vi "KeyDown.vi"(6 "PlatMods":T9, 7 "Type":T1, 8 "error in (no error)":errorcluster, 9 "VKey":T10, 10 "Char":i16, 11 "Data in":T2={"Class"={"Ants"=refnum, "Layer"=refnum, "Templates"=refnum, "Icon"=refnum, "Glyph"=refnum, "Settings"=refnum, "Tools"=refnum, "History"=refnum}, "Ref"={"Add Layer"=refnum, "Remove Layer"=refnum, "Line Text"=[], "Body Text Spec"=refnum, "DNL_Font"=refnum, "glyph path str"=refnum, "templates path str"=refnum, "Arrow Up"=refnum, "Arrow Down"=refnum, "IE VI Ref"=refnum, "Glyphs tree"=refnum, "Templates tree"=refnum, "Layer Icon Text"=refnum, "Layer Template"=refnum, "Body Text"=refnum, "Search Templates"=refnum, "TextMarker"=refnum, "Tab Control"=refnum, "Search Glyphs"=refnum, "Line Color"=refnum, "DNL_Glyphs []"=refnum, "Fill Color"=refnum, "Tools"=refnum, "Icon"=refnum, "Preview"=refnum, "Ants"=refnum, "Terminals"=refnum, "menu reference"=refnum, "LayerNames"=[], "GlyphLoadAnimation"=refnum, "TemplateLoadAnimation"=refnum, "refreshGlyphs"=refnum, "refreshTemplates"=refnum}, "Support"={"AntsRect"={"left"=0, "top"=0, "right"=0, "bottom"=0}, "Mouse Move Coords"={"Horizontal"=0, "Vertical"=0}, "Mouse Down Coords"={"Horizontal"=0, "Vertical"=0}, "Temp Coord"={"Horizontal"=0, "Vertical"=0}, "Action"=enum."Default", "Edge Color"=4914962, "Fill Color"=16860, "Mouse Down?"=FALSE, "Draft Mode?"=FALSE, "Temp Icon"=bytes[3102], "CTRL Pressed"=FALSE, "Move Selection?"=FALSE, "AntsRect Orig"={"left"=0, "top"=0, "right"=0, "bottom"=0}, "Text"="", "TM Set?"=FALSE, "Mouse inside icon?"=FALSE, "Tool (old value)"=0, "Pencil Move Color"=0, "Swap Colors?"=FALSE, "Shift pressed?"=FALSE}}) -> (0 "error out":errorcluster, 1 "Discard?":bool, 3 "Data out":T2={"Class"={"Ants"=refnum, "Layer"=refnum, "Templates"=refnum, "Icon"=refnum, "Glyph"=refnum, "Settings"=refnum, "Tools"=refnum, "History"=refnum}, "Ref"={"Add Layer"=refnum, "Remove Layer"=refnum, "Line Text"=[], "Body Text Spec"=refnum, "DNL_Font"=refnum, "glyph path str"=refnum, "templates path str"=refnum, "Arrow Up"=refnum, "Arrow Down"=refnum, "IE VI Ref"=refnum, "Glyphs tree"=refnum, "Templates tree"=refnum, "Layer Icon Text"=refnum, "Layer Template"=refnum, "Body Text"=refnum, "Search Templates"=refnum, "TextMarker"=refnum, "Tab Control"=refnum, "Search Glyphs"=refnum, "Line Color"=refnum, "DNL_Glyphs []"=refnum, "Fill Color"=refnum, "Tools"=refnum, "Icon"=refnum, "Preview"=refnum, "Ants"=refnum, "Terminals"=refnum, "menu reference"=refnum, "LayerNames"=[], "GlyphLoadAnimation"=refnum, "TemplateLoadAnimation"=refnum, "refreshGlyphs"=refnum, "refreshTemplates"=refnum}, "Support"={"AntsRect"={"left"=0, "top"=0, "right"=0, "bottom"=0}, "Mouse Move Coords"={"Horizontal"=0, "Vertical"=0}, "Mouse Down Coords"={"Horizontal"=0, "Vertical"=0}, "Temp Coord"={"Horizontal"=0, "Vertical"=0}, "Action"=enum."Default", "Edge Color"=4914962, "Fill Color"=16860, "Mouse Down?"=FALSE, "Draft Mode?"=FALSE, "Temp Icon"=bytes[3102], "CTRL Pressed"=FALSE, "Move Selection?"=FALSE, "AntsRect Orig"={"left"=0, "top"=0, "right"=0, "bottom"=0}, "Text"="", "TM Set?"=FALSE, "Mouse inside icon?"=FALSE, "Tool (old value)"=0, "Pencil Move Color"=0, "Swap Colors?"=FALSE, "Shift pressed?"=FALSE}})   [LabVIEW 2020]
uses:
  Class/Ants/Ants.lvclass
  Class/FakedArray/FakedArray.lvclass
  vi.lib/LabVIEW Icon API/lv_icon/Classes/Icon/Icon.lvclass
  Class/Icon Library/Glyph.lvclass
  Class/Settings/Settings.lvclass
  Class/Tools/Tools Paint.lvclass
  lv_icon.lvlib
  <vilib>/Utility/miscctls.llb/LVPoint32TypeDef.ctl
  <vilib>/event_ctls.llb/lveventtype.ctl
  Controls/SupportClass_Action.ctl
  <vilib>/event_ctls.llb/eventvkey.ctl
  Controls/Support Cluster.ctl
  Controls/References Cluster.ctl
  Controls/IE Classes.ctl
  Controls/Global Data.ctl
  vi.lib/LabVIEW Icon API/lv_icon/Controls/IEColor.ctl
  History/History/History.lvclass
panel:
  in  "Layer name":string="Clipboard"
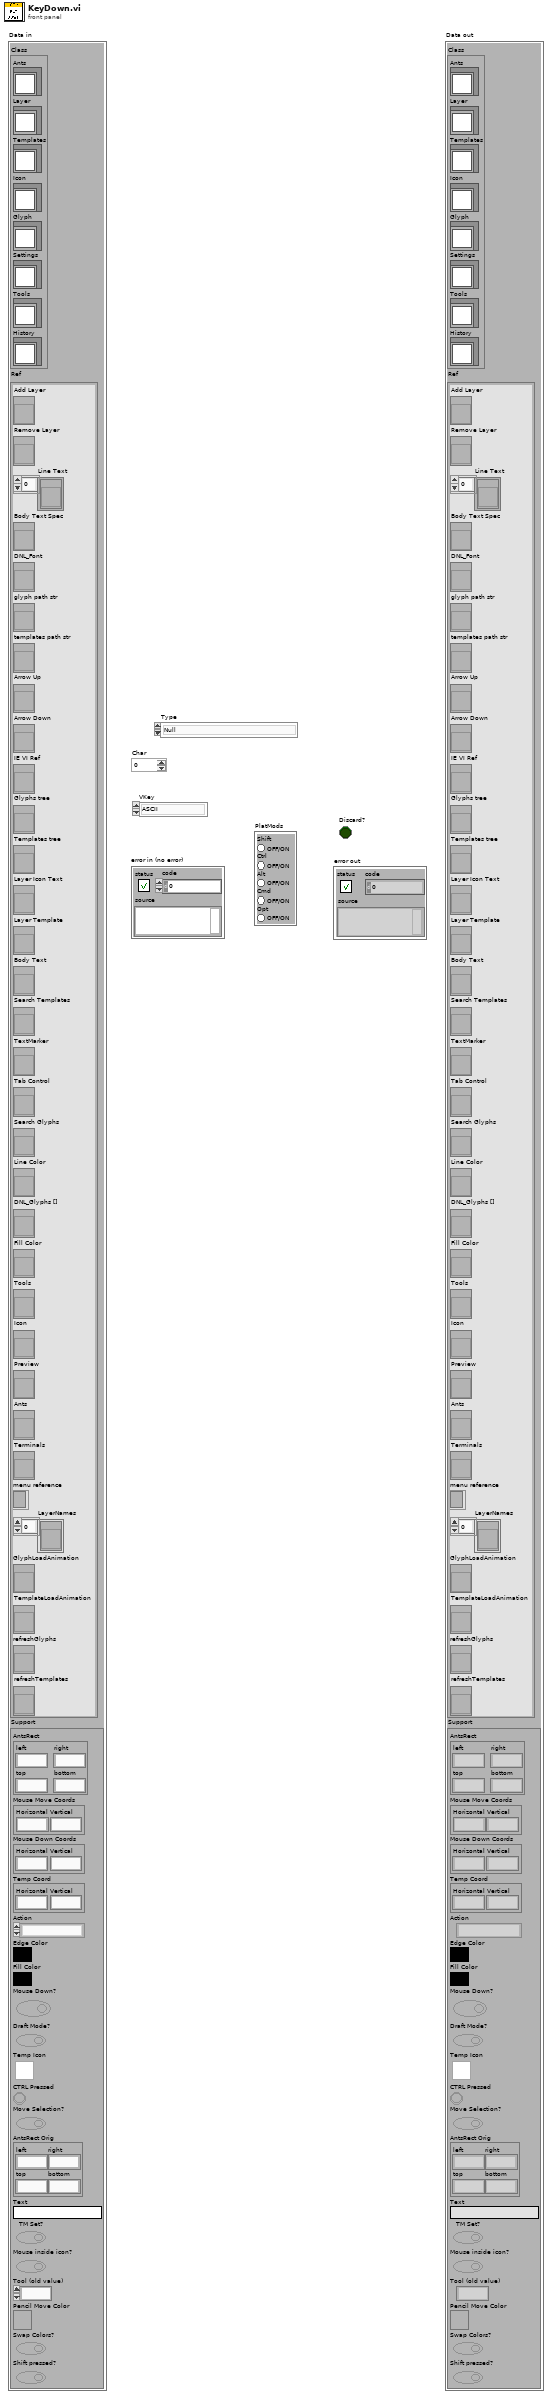
[diagram p1: front panel]
types:
  T1 = typedef "lveventtype.ctl" = enum32{"Null", "Timeout", "Annotation Menu Selection", "Annotation Menu Selection?", "App Instance Close", "App Instance Close?", "Autoscale Range Change", "Bookmark Info Change", "Cell Edit", "Cell Edit?", "Cursor Grab", "Cursor Grab?", "Cursor Menu Selection", "Cursor Menu Selection?", "Cursor Move", "Cursor Release", "Data Change", "Direction Change", "Display State Change", "Drag Ended", "Drag Enter", "Drag Leave", "Drag Over", "Drag Source Update", "Drag Starting", "Drag Starting?", "Drop", "Exec State Change", "Key Down", "Key Down?", "Key Repeat", "Key Repeat?", "Key Up", "Listbox Double Click", "Menu Activation?", "Menu Selection (App)", "Menu Selection? (App)", "Menu Selection (User)", "Mouse Down", "Mouse Down?", "Mouse Enter", "Mouse Leave", "Mouse Move", "Mouse Up", "Mouse Wheel", "NI Security User Change (App)", "Pane Size", "Panel Close", "Panel Close?", "Panel Resize", "Plot Attribute Change", "Scale Range Change", "Shortcut Menu Activation?", "Shortcut Menu Selection (App)", "Shortcut Menu Selection? (App)", "Shortcut Menu Selection (User)", "Tree Double Click", "Tree Drag", "Tree Drag?", "Tree Drop", "Tree Drop?", "Tree Item Close", "Tree Item Close?", "Tree Item Open", "Tree Item Open?", "URL Change?", "User Event", "Value Change"}
  T2 = typedef "lv_icon.lvlib/Global Data.ctl" = cluster{"Class":T3, "Ref":T4, "Support":T5}
  T3 = typedef "lv_icon.lvlib/IE Classes.ctl" = cluster{"Ants":refnum<class "Ants.lvclass">, "Layer":refnum<class "FakedArray.lvclass">, "Templates":refnum<class "FakedArray.lvclass">, "Icon":refnum<class "Icon.lvclass">, "Glyph":refnum<class "Glyph.lvclass">, "Settings":refnum<class "Settings.lvclass">, "Tools":refnum<class "Tools Paint.lvclass">, "History":refnum<class "History.lvclass">}
  T4 = typedef "lv_icon.lvlib/References Cluster.ctl" = cluster{"Add Layer":refnum<vi>, "Remove Layer":refnum<vi>, "Line Text":refnum<vi>[], "Body Text Spec":refnum<vi>, "DNL_Font":refnum<vi>, "glyph path str":refnum<vi>, "templates path str":refnum<vi>, "Arrow Up":refnum<vi>, "Arrow Down":refnum<vi>, "IE VI Ref":refnum<vi>, "Glyphs tree":refnum<vi>, "Templates tree":refnum<vi>, "Layer Icon Text":refnum<vi>, "Layer Template":refnum<vi>, "Body Text":refnum<vi>, "Search Templates":refnum<vi>, "TextMarker":refnum<vi>, "Tab Control":refnum<vi>, "Search Glyphs":refnum<vi>, "Line Color":refnum<vi>, "DNL_Glyphs []":refnum<vi>, "Fill Color":refnum<vi>, "Tools":refnum<vi>, "Icon":refnum<vi>, "Preview":refnum<vi>, "Ants":refnum<vi>, "Terminals":refnum<vi>, "menu reference":refnum<k9>, "LayerNames":refnum<vi>[], "GlyphLoadAnimation":refnum<vi>, "TemplateLoadAnimation":refnum<vi>, "refreshGlyphs":refnum<vi>, "refreshTemplates":refnum<vi>}
  T5 = typedef "lv_icon.lvlib/Support Cluster.ctl" = cluster{"AntsRect":cluster{"left":i16, "top":i16, "right":i16, "bottom":i16}, "Mouse Move Coords":T6, "Mouse Down Coords":T6, "Temp Coord":T6, "Action":T7, "Edge Color":T8, "Fill Color":T8, "Mouse Down?":bool, "Draft Mode?":bool, "Temp Icon":picture, "CTRL Pressed":bool, "Move Selection?":bool, "AntsRect Orig":cluster{"left":i16, "top":i16, "right":i16, "bottom":i16}, "Text":string, "TM Set?":bool, "Mouse inside icon?":bool, "Tool (old value)":u32, "Pencil Move Color":u32, "Swap Colors?":bool, "Shift pressed?":bool}
  T6 = typedef "LVPoint32TypeDef.ctl" = cluster{"Horizontal":i32, "Vertical":i32}
  T7 = typedef "SupportClass_Action.ctl" = enum16{"Default", "Move Selection", "Glyph Library", "Tool"}
  T8 = typedef "IEColor.ctl" = u32
  T9 = cluster{"Shift":bool, "Ctrl":bool, "Alt":bool, "Cmd":bool, "Opt":bool}
  T10 = typedef "eventvkey.ctl" = enum16{"ASCII", "Enter", "Return", "Shift", "Ctrl", "Alt", "Cmd", "Opt", "Caps", "NumLock", "Clear", "Break", "Up", "Down", "Left", "Right", "Insert", "Delete", "Home", "End", "PageUp", "PageDown", "Escape", "Help", "Pause", "ScrollLock", "F1", "F2", "F3", "F4", "F5", "F6", "F7", "F8", "F9", "F10", "F11", "F12", "F13", "F14", "F15", "F16", "F17", "F18", "F19", "F20", "F21", "F22", "F23", "F24", "Play", "VolumeUp", "VolumeDown", "Mute", "Two Byte Char"}
  T11 = cluster{"left":i16, "top":i16, "right":i16, "bottom":i16}
  T12 = enum32{"Pencil", "Line", "Dropper", "Fill", "Rectangle", "Filled Rectangle", "Ellipse", "Filled Ellipse", "Eraser", "Text", "Select", "Move"}
  T13 = typedef "Graphic.ctl" = cluster{"Rectangle":cluster{"left":i16, "top":i16, "right":i16, "bottom":i16}, "Path":path, "Image":picture, "Filter":string, "FileName":string}
  T14 = cluster{"left":i16, "top":i16, "bottom":i16, "right":i16}
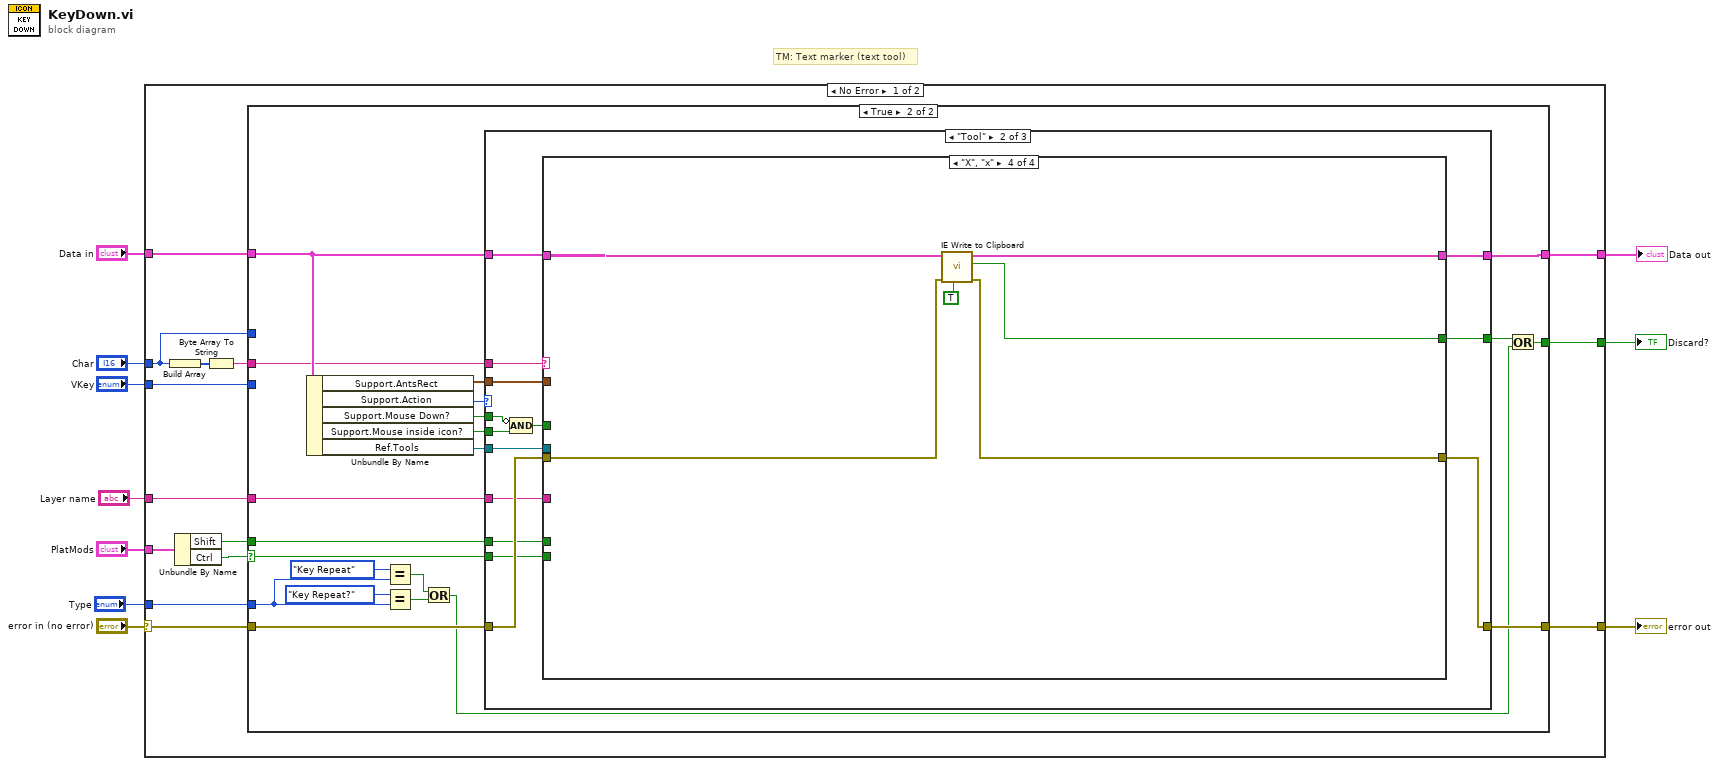
[diagram p0: block diagram]
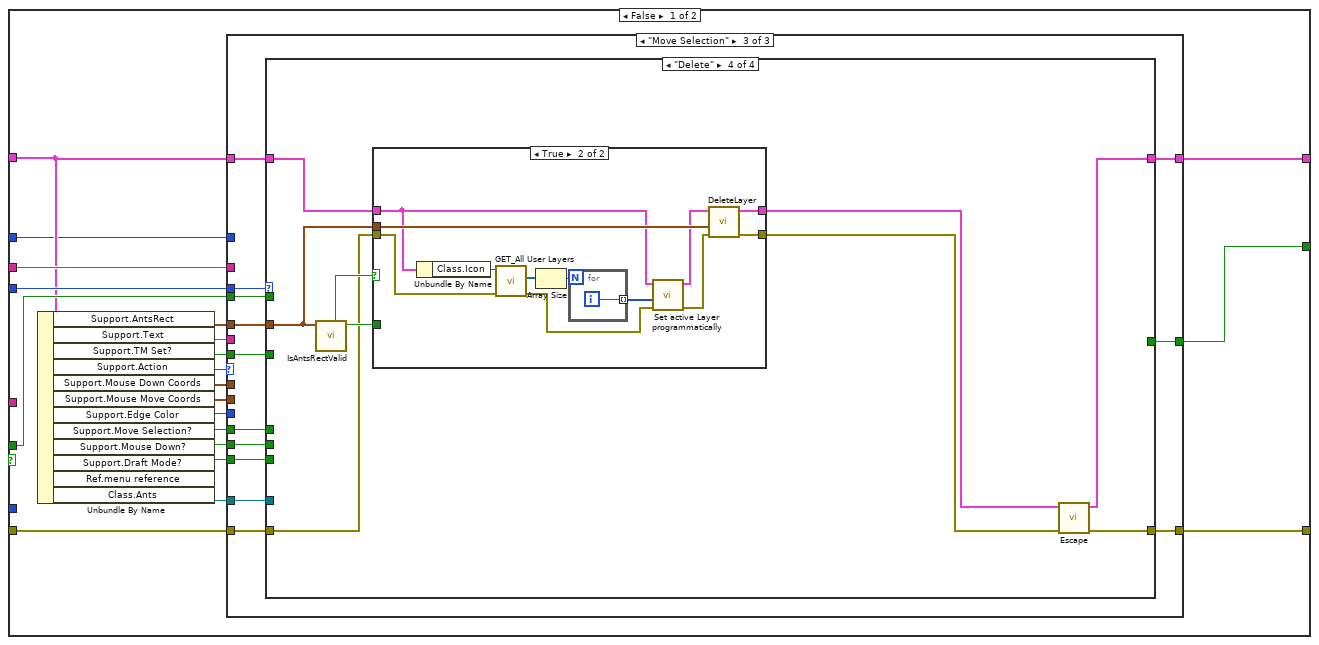
[diagram p2: hidden frame]
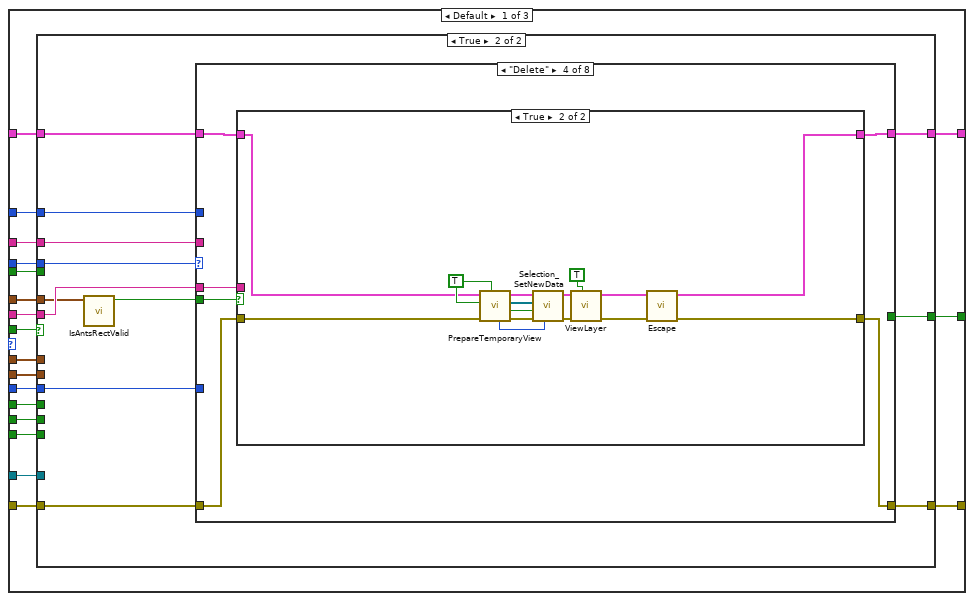
[diagram p3: hidden frame]
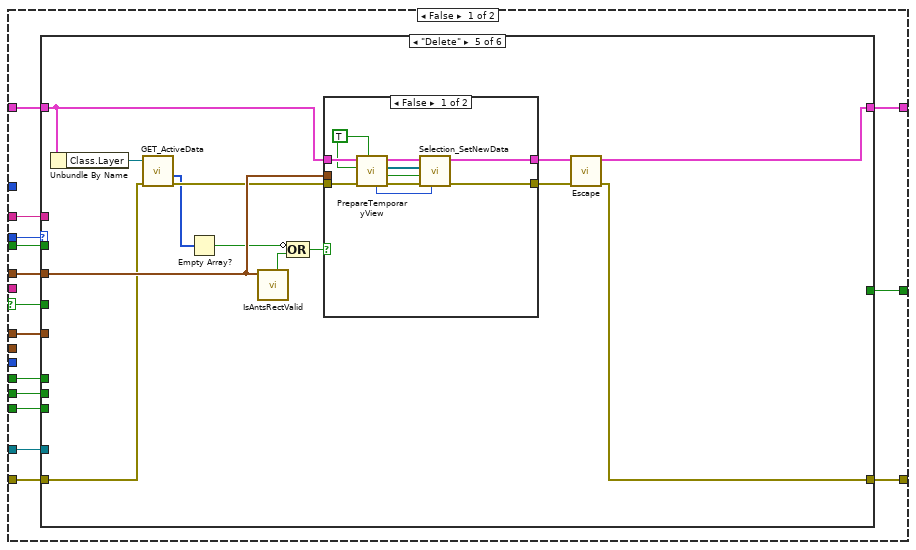
[diagram p4: hidden frame]
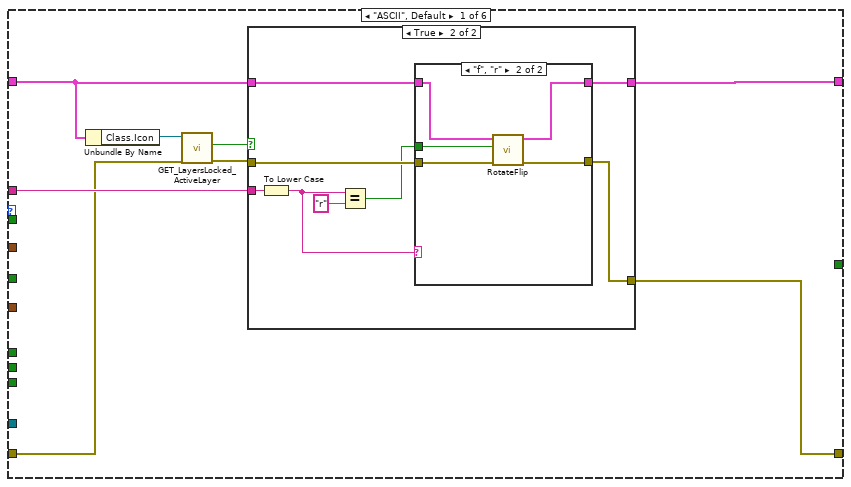
[diagram p5: hidden frame]
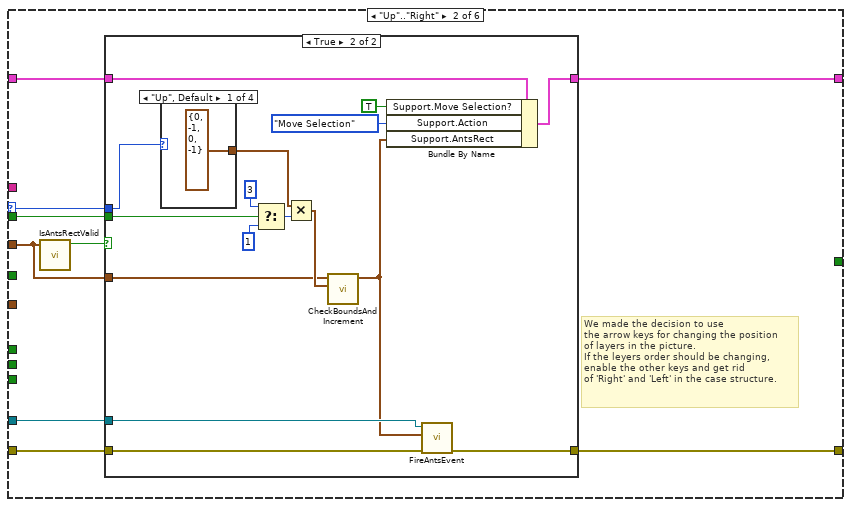
[diagram p8: hidden frame]
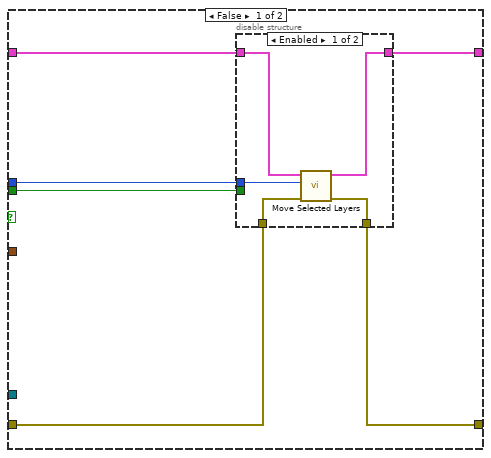
[diagram p9: hidden frame]
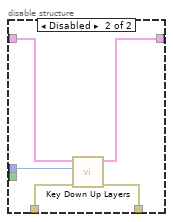
[diagram p10: hidden frame]
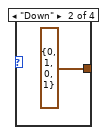
[diagram p11: hidden frame]
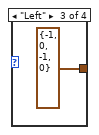
[diagram p12: hidden frame]
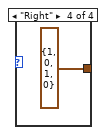
[diagram p13: hidden frame]
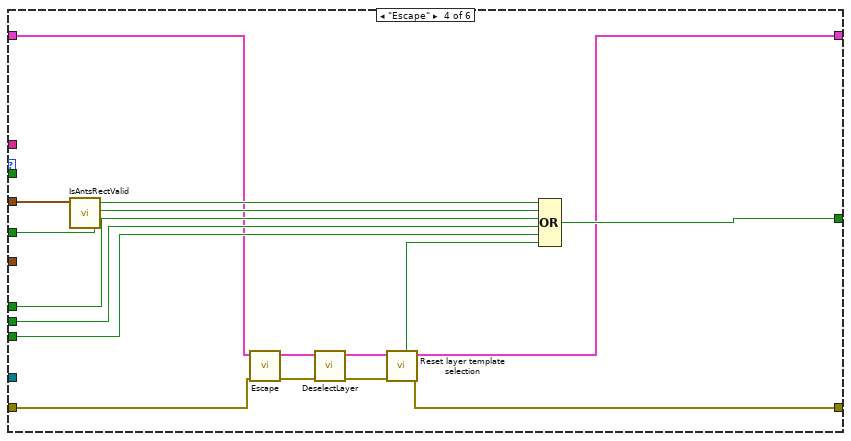
[diagram p15: hidden frame]
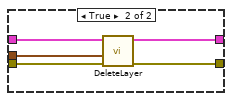
[diagram p16: hidden frame]
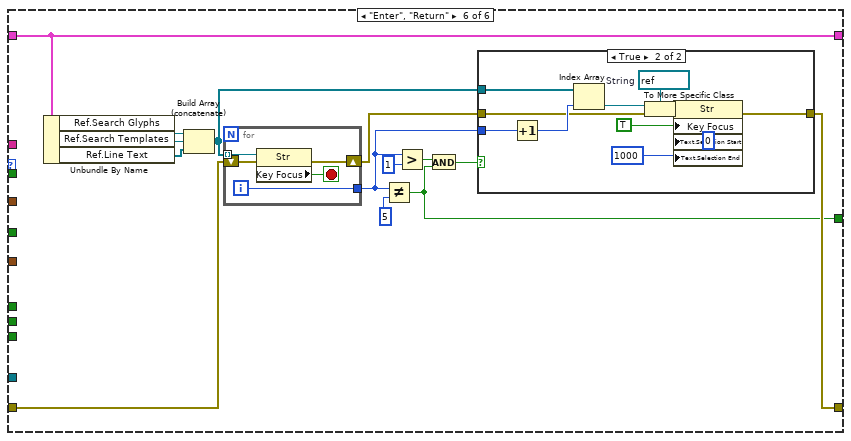
[diagram p17: hidden frame]
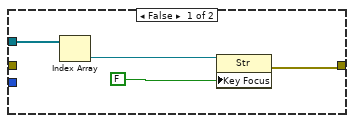
[diagram p18: hidden frame]
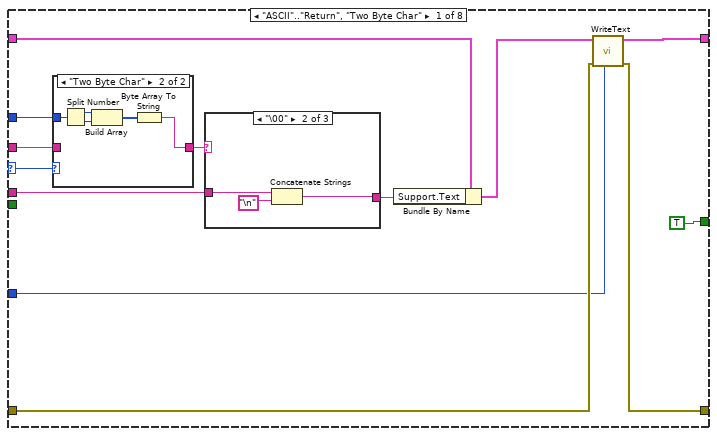
[diagram p19: hidden frame]
diagram:
  # "TM: Text marker (text tool)"
  n1 = case shown="No Error" "error in (no error)" {
    selector: "error in (no error)" -> [w17 w699]
    tunnel: [w21 w699] -> w9
    tunnel: "VKey" -> [w24 _]
    tunnel: "Char" -> [w12 _]
    tunnel: "PlatMods" -> [w20 _]
    tunnel: [w18 _] -> w5
    tunnel: "Data in" -> [w15 w698]
    tunnel: [w14 w698] -> w3
    tunnel: "Type" -> [w13 _]
    tunnel: "Layer name" -> [w11 _]
    frame No Error {
      n2 = Build Array(w12) -> (w23:i16[])
      n3 = Unbundle By Name(w20) -> ("Shift"=w16:bool, "Ctrl"=w19:bool)
      n4 = Byte Array To String(unsigned byte array=w23) -> (string=w22:string)
      n5 = case shown="True" w19 {
        selector: w19 -> [_ w490]
        tunnel: w24 -> [w44 _]
        tunnel: w22 -> [w43 w488]
        tunnel: [w28 w500] -> w21
        tunnel: [w32 w487] -> w18
        tunnel: w17 -> [w30 w503]
        tunnel: w16 -> [w31 w491]
        tunnel: w15 -> [w29 w502]
        tunnel: [w26 w501] -> w14
        tunnel: w13 -> [_ w495]
        tunnel: w12 -> [w25 _]
        tunnel: w11 -> [_ w485]
        frame False {
          n6 = Unbundle By Name(w29) -> ("Support.AntsRect"=w37:T11, "Support.Text"=w40:string, "Support.TM Set?"=w41:bool, "Support.Action"=w42:T7, "Support.Mouse Down Coords"=w39:T6, "Support.Mouse Move Coords"=w36:T6, "Support.Edge Color"=w38:T8, "Support.Move Selection?"=w35:bool, "Support.Mouse Down?"=w34:bool, "Support.Draft Mode?"=w33:bool, "Class.Ants"=w27:refnum<class "Ants.lvclass">)  [unwired: 1 out]
          n7 = case shown="\"Move Selection\"" w42 {
            tunnel: w44 -> [w63 w336 w403]
            tunnel: w43 -> [w58 w335 _]
            tunnel: w30 -> [w61 w334 w405]
            tunnel: [w62 w333 w404] -> w28
            tunnel: w41 -> [w60 w331 w401]
            tunnel: w40 -> [w59 _ _]
            tunnel: w39 -> [w57 _ _]
            tunnel: w38 -> [w56 _ _]
            tunnel: w37 -> [w55 w332 w402]
            tunnel: w36 -> [w54 w324 _]
            tunnel: w35 -> [w53 w330 w400]
            tunnel: w34 -> [w52 w329 w399]
            tunnel: w33 -> [w51 w328 w398]
            tunnel: [w50 w327 w397] -> w32
            tunnel: w31 -> [w49 _ w393]
            tunnel: w29 -> [w48 w326 w396]
            tunnel: [w47 w325 w395] -> w26
            tunnel: w27 -> [w45 _ w394]
            tunnel: w25 -> [w46 _ _]
            frame Default {
              n8 = case shown="True" w60 {
                selector: w60 -> [w69 _]
                tunnel: w63 -> [w77 w240]
                tunnel: [w76 w239] -> w62
                tunnel: w61 -> [w78 w238]
                tunnel: w59 -> [_ w237]
                tunnel: w58 -> [w75 w236]
                tunnel: w57 -> [w73 _]
                tunnel: w56 -> [_ w233]
                tunnel: w55 -> [w74 w235]
                tunnel: w54 -> [_ _]
                tunnel: w53 -> [w72 _]
                tunnel: w52 -> [w71 _]
                tunnel: w51 -> [w70 _]
                tunnel: [w68 w232] -> w50
                tunnel: w49 -> [w67 _]
                tunnel: w48 -> [w66 w231]
                tunnel: [w65 w230] -> w47
                tunnel: w46 -> [_ w229]
                tunnel: w45 -> [w64 _]
                frame False {
                  n9 = case shown="\"Delete\"" w77 {
                    selector: w77 -> [_ w110 _ _ _ _]
                    tunnel: w78 -> [w82 w112 w150 w166 w173 w207]
                    tunnel: [w85 w111 w150 w163 w179 w204] -> w76
                    tunnel: w75 -> [w86 _ _ _ _ _]
                    tunnel: w74 -> [_ w105 _ w161 w176 _]
                    tunnel: w73 -> [_ _ _ _ _ _]
                    tunnel: w72 -> [_ _ _ w159 _ _]
                    tunnel: w71 -> [_ _ _ w158 _ _]
                    tunnel: w70 -> [_ _ _ w157 _ _]
                    tunnel: w69 -> [_ _ _ w160 _ _]
                    tunnel: [_ _ _ w156 _ w196] -> w68
                    tunnel: w67 -> [_ w109 _ _ _ _]
                    tunnel: w66 -> [w84 w108 w149 w154 w174 w208]
                    tunnel: [w83 w107 w149 w151 w178 w208] -> w65
                    tunnel: w64 -> [_ w104 _ _ _ _]
                    frame "ASCII", Default {
                      n10 = Unbundle By Name(w84) -> ("Class.Icon"=w80:refnum<class "Icon.lvclass">)
                      n11 = call-dynamic "GET_LayersLocked_ActiveLayer.vi"("error in (no error)"=w82, "Icon.lvclass in"=w80) -> ("error out"=w81:errorcluster, "Layers Locked?"=w79:bool)  [unwired: 8 out]
                      n12 = case shown="True" w79 {
                        tunnel: w86 -> [_ w93]
                        tunnel: w81 -> [w88 w96]
                        tunnel: [w88 w95] -> w85
                        tunnel: w84 -> [w87 w90]
                        tunnel: [w87 w89] -> w83
                        frame False {
                        }
                        frame True {
                          n13 = To Lower Case(string=w93) -> (all lower case string=w91:string)
                          n14 = Equal?(x=w91, y="r") -> (x = y?=w92:bool)
                          n15 = case shown="\"f\", \"r\"" w91 {
                            tunnel: w96 -> [w98 w103]
                            tunnel: [w98 w101] -> w95
                            tunnel: w92 -> [_ w102]
                            tunnel: w90 -> [w97 w100]
                            tunnel: [w97 w99] -> w89
                            frame Default {
                            }
                            frame "f", "r" {
                              n16 = call "RotateFlip.vi"("error in"=w103, "Rotate"=w102, "Data in"=w100) -> ("error out"=w101:errorcluster, "Data out"=w99:T2)  [unwired: 3 in, 4 out]
                            }
                          }
                        }
                      }
                    }
                    frame "Up".."Right" {
                      # "We made the decision to use\nthe arrow keys for changing the position\nof layers in the picture.\nIf the leyers order should be changing,\nenable the other keys and get rid\nof 'Right' and 'Left' in the case structure."
                      n17 = call "IsAntsRectValid.vi"("AntsRect"=w105) -> ("Valid?"=w106:bool)  [unwired: 10 out]
                      n18 = case shown="True" w106 {
                        tunnel: w112 -> [w118 w129]
                        tunnel: [w117 w133] -> w111
                        tunnel: w110 -> [w116 w135]
                        tunnel: w109 -> [w115 w134]
                        tunnel: w108 -> [w114 w143]
                        tunnel: [w113 w141] -> w107
                        tunnel: w105 -> [_ w131]
                        tunnel: w104 -> [_ w132]
                        frame False {
                          n19 = disable-structure shown="Enabled" {
                            disable-tunnel: w118 -> [w121 w126]
                            disable-tunnel: [w120 w125] -> w117
                            disable-tunnel: w116 -> [w119 w124]
                            disable-tunnel: w115 -> [_ _]
                            disable-tunnel: w114 -> [w123 w128]
                            disable-tunnel: [w122 w127] -> w113
                            frame Enabled {
                              n20 = call "Move Selected Layers.vi"("error in"=w121, "VKey"=w119, "Data in"=w123) -> ("error out"=w120:errorcluster, "Data out"=w122:T2)  [unwired: 1 in, 6 out]
                            }
                            frame Disabled {
                              n21 = call "Key Down Up Layers.vi"("error in"=w126, "VKey"=w124, "Data in"=w128) -> ("error out"=w125:errorcluster, "Data out"=w127:T2)  [unwired: 1 in, 6 out]
                            }
                          }
                        }
                        frame True {
                          n22 = case shown="\"Up\", Default" w135 {
                            tunnel: [T11 {"left"=0, "top"=-1, "right"=0, "bottom"=-1} ("y") T11 {"left"=0, "top"=1, "right"=0, "bottom"=1} ("y") T11 {"left"=-1, "top"=0, "right"=-1, "bottom"=0} ("y") T11 {"left"=1, "top"=0, "right"=1, "bottom"=0} ("y")] -> w139
                            frame "Up", Default {
                            }
                            frame "Down" {
                            }
                            frame "Left" {
                            }
                            frame "Right" {
                            }
                          }
                          n23 = Select(t=i16 3 ("left"), s=w134, f=i16 1 ("left")) -> (s? t:f=w136:i16)
                          n24 = Multiply(x=w139, y=w136) -> (x*y=w144:T11)
                          n25 = call "CheckBoundsAndIncrement.vi"("Increment"=w144, "Rectangle In"=w131) -> ("Rectangle Out"=w130:T11)  [unwired: 9 in]
                          n26 = Bundle By Name(cluster=w143, "Support.Move Selection?"=TRUE, "Support.Action"=SupportClass_Action."Move Selection", "Support.AntsRect"=w130) -> (w141:T2)
                          n27 = call "FireAntsEvent.vi"("error in (no error)"=w129, "Rectangle (default: deselect)"=w130, "Ants in"=w132) -> ("error out"=w133:errorcluster)  [unwired: 1 in, 7 out]
                        }
                      }
                    }
                    frame "Shift" {
                    }
                    frame "Escape" {
                      n28 = call "IsAntsRectValid.vi"("AntsRect"=w161) -> ("Valid?"=w162:bool)  [unwired: 10 out]
                      n29 = call "Escape.vi"("error in"=w166, "Data in"=w154) -> ("error out"=w165:errorcluster, "Data out"=w153:T2)  [unwired: 8 out]
                      n30 = call "DeselectLayer.vi"("error in (no error)"=w165, "Data in"=w153) -> ("error out"=w164:errorcluster, "Data out"=w152:T2)  [unwired: 8 out]
                      n31 = call "Reset layer template selection.vi"("error in (no error)"=w164, "Data in"=w152) -> ("error out"=w163:errorcluster, "Data out"=w151:T2, "Layers selected?"=w155:bool)  [unwired: 1 in, 6 out]
                      n32 = Compound Arithmetic op=OR(w162, w160, w159, w158, w157, w155) -> (w156:bool)
                    }
                    frame "Delete" {
                      n33 = Unbundle By Name(w174) -> ("Class.Layer"=w175:refnum<class "FakedArray.lvclass">)
                      n34 = call-dynamic "GET_ActiveData.vi"("error in (no error)"=w173, "FakedArray in"=w175) -> ("error out"=w172:errorcluster, "Active Data []"=w171:i32[])  [unwired: 4 in, 4 out]
                      n35 = Empty Array?(array=w171) -> (empty?=w169:bool)
                      n36 = call "IsAntsRectValid.vi"("AntsRect"=w176) -> ("Max. Rect size?"=w170:bool)  [unwired: 10 out]
                      n37 = Compound Arithmetic op=OR(invert w169, w170) -> (w168:bool)
                      n38 = case shown="False" w168 {
                        tunnel: w174 -> [w189 w194]
                        tunnel: [w188 w192] -> w177
                        tunnel: [w187 w193] -> w167
                        tunnel: w172 -> [w180 w191]
                        tunnel: w176 -> [_ w190]
                        frame False {
                          w186 = TRUE ("Delete Selected Area?")
                          n39 = call "PrepareTemporaryView.vi"("Delete Selected Area?"=w186, "error in (no error)"=w180, "Valid Selection?"=w186, "Data in"=w189) -> ("error out"=w183:errorcluster, "Highlighted?"=w184:bool, "All Layers out"=w185:refnum<class "Layer.lvclass">[], "Data out"=w181:T2, "#Active Layer"=w182:i32)  [unwired: 1 in, 2 out]
                          n40 = call "Selection_SetNewData.vi"("#Active Layer"=w182, "error in"=w183, "Highlighted?"=w184, "All Layers In"=w185, "Data in"=w181) -> ("error out"=w188:errorcluster, "Data out"=w187:T2)  [unwired: 1 in, 3 out]
                        }
                        frame True {
                          n41 = call "DeleteLayer.vi"("error in"=w191, "AntsRect"=w190, "Data in"=w194) -> ("error out"=w192:errorcluster, "Data out"=w193:T2)  [unwired: 5 out]
                        }
                      }
                      n42 = call "Escape.vi"("error in"=w177, "Data in"=w167) -> ("error out"=w179:errorcluster, "Data out"=w178:T2)  [unwired: 8 out]
                    }
                    frame "Enter", "Return" {
                      n43 = Unbundle By Name(w208) -> ("Ref.Search Glyphs"=w200:refnum<vi>, "Ref.Search Templates"=w201:refnum<vi>, "Ref.Line Text"=w203:refnum<vi>[])
                      n44 = Build Array (concatenate)(w200, w201, w203) -> (w202:refnum<vi>[])
                      n45 = for {
                        tunnel: w202 -> [w228] mode=indexing
                        shift-right: [w227] -> w205
                        shift-left: w207 -> [w226]
                        tunnel: [w225] -> w199
                        i -> [w225]
                        stop <- w224 stop-if-true
                        n46 = property class="Str"(reference=w228, error in=w226) -> (error out=w227:errorcluster, "Key Focus"=w224:bool)  [unwired: 1 out]
                      }
                      n47 = Not Equal?(x=w199, y=5) -> (x != y?=w196:bool)
                      n48 = Greater?(x=w199, y=1) -> (0:w197:bool)
                      n49 = And(x=w197, y=w196) -> (x .and. y?=w195:bool)
                      n50 = case shown="True" w195 {
                        tunnel: w199 -> [_ w222]
                        tunnel: w202 -> [w212 w223]
                        tunnel: w205 -> [_ w219]
                        tunnel: [w209 w217] -> w204
                        frame False {
                          n51 = Index Array(array=w212) -> (element=w211:refnum<vi>)  [unwired: 1 in]
                          n52 = property class="Str"(reference=w211, "Key Focus"=FALSE) -> (error out=w209:errorcluster)  [unwired: 1 in, 1 out]
                        }
                        frame True {
                          w213 = refnum<vi> refnum  # String
                          n53 = Increment(x=w222) -> (x+1=w221:i32)
                          n54 = Index Array(array=w223, index=w221) -> (element=w220:refnum<vi>)
                          n55 = To More Specific Class(target class=w213, reference=w220) -> (specific class reference=w214:refnum<vi>)  [unwired: 1 in, 1 out]
                          n56 = property class="Str"(reference=w214, error in=w219, "Key Focus"=TRUE, "Text.Selection Start"=u32 0 ("Text.Selection:Start"), "Text.Selection End"=u32 1000 ("Text.Selection:End")) -> (error out=w217:errorcluster)  [unwired: 1 out]
                        }
                      }
                    }
                  }
                }
                frame True {
                  n57 = call "IsAntsRectValid.vi"("AntsRect"=w235) -> ("Valid?"=w234:bool)  [unwired: 10 out]
                  n58 = case shown="\"Delete\"" w240 {
                    selector: w240 -> [w244 _ _ _ _ _ _ _]
                    tunnel: [w251 w273 w276 w280 w303 w309 w315 w321] -> w239
                    tunnel: w238 -> [w252 w274 w276 w281 w304 w310 w316 w322]
                    tunnel: w237 -> [w253 _ _ w282 _ _ _ _]
                    tunnel: w236 -> [w242 _ _ _ _ _ _ _]
                    tunnel: w233 -> [w250 _ _ _ w305 w311 w317 w323]
                    tunnel: w234 -> [_ _ _ w279 _ _ _ _]
                    tunnel: [TRUE TRUE _ _ _ _ _ _] -> w232
                    tunnel: w231 -> [w245 w271 w275 w278 w302 w307 w314 w320]
                    tunnel: [w248 w270 w275 w277 w300 w306 w313 w318] -> w230
                    tunnel: w229 -> [w241 _ _ _ _ _ _ _]
                    frame "ASCII".."Return", "Two Byte Char" {
                      n59 = case shown="\"Two Byte Char\"" w244 {
                        tunnel: [w254 w255] -> w243
                        tunnel: w242 -> [w254 _]
                        tunnel: w241 -> [_ w259]
                        frame "ASCII", Default {
                        }
                        frame "Two Byte Char" {
                          n60 = Split Number(x=w259) -> (hi(x)=w257:u8, lo(x)=w258:u8)
                          n61 = Build Array(w257, w258) -> (w256:u8[])
                          n62 = Byte Array To String(unsigned byte array=w256) -> (string=w255:string)
                        }
                      }
                      n63 = case shown="\"\\00\"" w243 {
                        selector: w243 -> [_ _ w267]
                        tunnel: w253 -> [w261 w266 w269]
                        tunnel: [w260 w265 w268] -> w247
                        frame "\b" {
                          n64 = String Length(string=w261) -> (length=w263:i32)
                          n65 = Decrement(x=w263) -> (x-1=w262:i32)
                          n66 = Search/Split String(string=w261, offset (0)=w262) -> (substring before match=w260:string)  [unwired: 3 out]
                        }
                        frame "\u0000\u0000" {
                          n67 = Concatenate Strings(w266, "\n") -> (w265:string)
                        }
                        frame Default {
                          n68 = Concatenate Strings(w269, w267) -> (w268:string)
                        }
                      }
                      n69 = Bundle By Name(cluster=w245, "Support.Text"=w247) -> (w246:T2)
                      n70 = call "WriteText.vi"("Text Color"=w250, "error in (no error)"=w252, "Data in"=w246) -> ("error out"=w251:errorcluster, "Data out"=w248:T2)  [unwired: 2 in, 5 out]
                    }
                    frame "Escape" {
                      n71 = call "Escape.vi"("error in"=w274, "Data in"=w271) -> ("error out"=w273:errorcluster, "Data out"=w270:T2)  [unwired: 8 out]
                    }
                    frame Default {
                    }
                    frame "Delete" {
                      n72 = case shown="True" w279 {
                        tunnel: w282 -> [_ _]
                        tunnel: w281 -> [w284 w292]
                        tunnel: [w284 w294] -> w280
                        tunnel: w278 -> [w283 w285]
                        tunnel: [w283 w289] -> w277
                        frame False {
                        }
                        frame True {
                          w299 = TRUE ("Delete Selected Area?")
                          n73 = call "PrepareTemporaryView.vi"("Delete Selected Area?"=w299, "error in (no error)"=w292, "Valid Selection?"=w299, "Data in"=w285) -> ("error out"=w295:errorcluster, "Highlighted?"=w297:bool, "All Layers out"=w298:refnum<class "Layer.lvclass">[], "Data out"=w291:T2, "#Active Layer"=w296:i32)  [unwired: 1 in, 2 out]
                          n74 = call "Selection_SetNewData.vi"("#Active Layer"=w296, "error in"=w295, "Highlighted?"=w297, "All Layers In"=w298, "Data in"=w291) -> ("error out"=w293:errorcluster, "Data out"=w290:T2)  [unwired: 1 in, 3 out]
                          n75 = call "ViewLayer.vi"("Add to Undo?"=TRUE, "error in (no error)"=w293, "Data in"=w290) -> ("error out"=w288:errorcluster, "Data out"=w287:T2)  [unwired: 2 in, 5 out]
                          n76 = call "Escape.vi"("error in"=w288, "Data in"=w287) -> ("error out"=w294:errorcluster, "Data out"=w289:T2)  [unwired: 8 out]
                        }
                      }
                    }
                    frame "Up" {
                      n77 = call "WriteText.vi"("Text Color"=w305, "error in (no error)"=w304, "Offset"=T6 {"Horizontal"=0, "Vertical"=-1} ("y"), "Data in"=w302) -> ("error out"=w303:errorcluster, "Data out"=w300:T2)  [unwired: 1 in, 5 out]
                    }
                    frame "Down" {
                      n78 = call "WriteText.vi"("Text Color"=w311, "error in (no error)"=w310, "Offset"=T6 {"Horizontal"=0, "Vertical"=1} ("y"), "Data in"=w307) -> ("error out"=w309:errorcluster, "Data out"=w306:T2)  [unwired: 1 in, 5 out]
                    }
                    frame "Left" {
                      n79 = call "WriteText.vi"("Text Color"=w317, "error in (no error)"=w316, "Offset"=T6 {"Horizontal"=-1, "Vertical"=0} ("y"), "Data in"=w314) -> ("error out"=w315:errorcluster, "Data out"=w313:T2)  [unwired: 6 out]
                    }
                    frame "Right" {
                      n80 = call "WriteText.vi"("Text Color"=w323, "error in (no error)"=w322, "Offset"=T6 {"Horizontal"=1, "Vertical"=0} ("y"), "Data in"=w320) -> ("error out"=w321:errorcluster, "Data out"=w318:T2)  [unwired: 6 out]
                    }
                  }
                }
              }
            }
            frame "Glyph Library" {
              n81 = case shown="\"Escape\"" w336 {
                tunnel: w334 -> [w341 w388 w391]
                tunnel: [w340 w387 w391] -> w333
                tunnel: w335 -> [w342 _ _]
                tunnel: w332 -> [_ w385 _]
                tunnel: w331 -> [_ w384 _]
                tunnel: w330 -> [_ w383 _]
                tunnel: w329 -> [_ w382 _]
                tunnel: w328 -> [_ w381 _]
                tunnel: [_ w380 _] -> w327
                tunnel: w326 -> [w339 w379 w390]
                tunnel: [w338 w377 w389] -> w325
                tunnel: w324 -> [w337 _ _]
                frame "ASCII", Default {
                  n82 = case shown="Default" w342 {
                    selector: w342 -> [_ w361]
                    tunnel: w341 -> [w344 w347]
                    tunnel: [w344 w346] -> w340
                    tunnel: w339 -> [w343 w351]
                    tunnel: [w343 w348] -> w338
                    tunnel: w337 -> [_ w345]
                    frame Default {
                    }
                    frame "F", "R", "f", "r" {
                      n83 = Unbundle By Name(w351) -> ("Class.Glyph"=w352:refnum<class "Glyph.lvclass">)
                      n84 = call-dynamic "GET_ActiveGlyph.vi"("error in (no error)"=w347, "Glyph.lvclass in"=w352) -> ("error out"=w364:errorcluster, "Path & Icon"=w366:T13, "Glyph.lvclass out"=w365:refnum<class "Glyph.lvclass">)  [unwired: 7 out]
                      n85 = Unbundle By Name(w366) -> ("Image"=w368:picture, "Rectangle"=w367:T11)
                      n86 = Equal?(x=w361, y="r") -> (x = y?=w358:bool)
                      n87 = Equal?(x=w361, y="R") -> (x = y?=w359:bool)
                      n88 = Or(x=w358, y=w359) -> (x .or. y?=w353:bool)
                      n89 = call "Rotate Flip Image.vi"("Rotate?"=w353, "rect"=w367, "Temp Icon In"=w368) -> ("rect out"=w356:T14, "Temp Icon Out"=w357:picture)  [unwired: 7 out]
                      n90 = case shown="False" w353 {
                        tunnel: w357 -> [w373 w375]
                        tunnel: w356 -> [w372 w374]
                        tunnel: [w371 w375] -> w355
                        tunnel: [w370 w374] -> w354
                        frame False {
                          n91 = call "Rotate Flip Image.vi"("Rotate?"=TRUE, "rect"=w372, "Temp Icon In"=w373) -> ("rect out"=w370:T14, "Temp Icon Out"=w371:picture)  [unwired: 7 out]
                        }
                        frame True {
                        }
                      }
                      n92 = Bundle By Name(cluster=w366, "Image"=w355, "Rectangle"=w354) -> (w363:T13)
                      n93 = call "TemporaryGlyphView.vi"("Mouse Coords Pic"=w345, "Path & Icon"=w363) -> ("icon out"=w349:picture)  [unwired: 9 out]
                      n94 = call-dynamic "SET_ActiveGlyph.vi"("error in (no error)"=w364, "Active Glyph"=w363, "Glyph in"=w365) -> ("error out"=w346:errorcluster, "Glyph out"=w350:refnum<class "Glyph.lvclass">)  [unwired: 7 out]
                      n95 = Bundle By Name(cluster=w351, "Class.Glyph"=w350, "Support.Temp Icon"=w349) -> (w348:T2)
                    }
                  }
                }
                frame "Escape" {
                  n96 = call "IsAntsRectValid.vi"("AntsRect"=w385) -> ("Valid?"=w386:bool)  [unwired: 10 out]
                  n97 = Compound Arithmetic op=OR(w386, w384, w383, w382, w381) -> (w380:bool)
                  n98 = call "Escape.vi"("error in"=w388, "Data in"=w379) -> ("error out"=w376:errorcluster, "Data out"=w378:T2)  [unwired: 8 out]
                  n99 = call "Reset layer template selection.vi"("error in (no error)"=w376, "Data in"=w378) -> ("error out"=w387:errorcluster, "Data out"=w377:T2)  [unwired: 1 in, 7 out]
                }
                frame "Ctrl" {
                  n100 = Bundle By Name(cluster=w390, "Support.CTRL Pressed"=TRUE ("CTRL Pressed")) -> (w389:T2)
                }
              }
            }
            frame "Move Selection" {
              n101 = case shown="\"Delete\"" w403 {
                selector: w403 -> [_ w412 _ _]
                tunnel: w405 -> [w407 w410 w444 w453]
                tunnel: [w407 w409 w437 w460] -> w404
                tunnel: w402 -> [_ w414 w451 w452]
                tunnel: w401 -> [_ _ w449 _]
                tunnel: w400 -> [_ _ w448 _]
                tunnel: w399 -> [_ _ w447 _]
                tunnel: w398 -> [_ _ w446 _]
                tunnel: [_ _ w445 _] -> w397
                tunnel: w396 -> [w406 w416 w441 w454]
                tunnel: [w406 w413 w438 w458] -> w395
                tunnel: w394 -> [_ w408 w443 _]
                tunnel: w393 -> [_ w411 _ _]
                frame "ASCII", Default {
                }
                frame "Up".."Right" {
                  n102 = call "IsAntsRectValid.vi"("AntsRect"=w414) -> ("Valid?"=w415:bool)  [unwired: 10 out]
                  n103 = case shown="True" w415 {
                    tunnel: w416 -> [w418 w432]
                    tunnel: w414 -> [_ w421]
                    tunnel: [w418 w431] -> w413
                    tunnel: w412 -> [_ w425]
                    tunnel: w411 -> [_ w429]
                    tunnel: w410 -> [w417 w419]
                    tunnel: [w417 w424] -> w409
                    tunnel: w408 -> [_ w423]
                    frame False {
                    }
                    frame True {
                      n104 = case shown="\"Up\", Default" w425 {
                        tunnel: [T11 {"left"=0, "top"=-1, "right"=0, "bottom"=-1} ("y") T11 {"left"=0, "top"=1, "right"=0, "bottom"=1} ("y") T11 {"left"=-1, "top"=0, "right"=-1, "bottom"=0} ("y") T11 {"left"=1, "top"=0, "right"=1, "bottom"=0} ("y")] -> w430
                        frame "Up", Default {
                        }
                        frame "Down" {
                        }
                        frame "Left" {
                        }
                        frame "Right" {
                        }
                      }
                      n105 = Select(t=i16 3 ("left"), s=w429, f=i16 1 ("left")) -> (s? t:f=w426:i16)
                      n106 = Multiply(x=w430, y=w426) -> (x*y=w422:T11)
                      n107 = call "CheckBoundsAndIncrement.vi"("Increment"=w422, "Rectangle In"=w421) -> ("Rectangle Out"=w420:T11)  [unwired: 9 in]
                      n108 = Bundle By Name(cluster=w432, "Support.AntsRect"=w420) -> (w431:T2)
                      n109 = call "FireAntsEvent.vi"("error in (no error)"=w419, "Rectangle (default: deselect)"=w420, "Ants in"=w423) -> ("error out"=w424:errorcluster)  [unwired: 1 in, 7 out]
                    }
                  }
                }
                frame "Escape" {
                  n110 = call "IsAntsRectValid.vi"("AntsRect"=w451) -> ("Valid?"=w450:bool)  [unwired: 10 out]
                  n111 = Compound Arithmetic op=OR(w450, w449, w448, w447, w446) -> (w445:bool)
                  n112 = call "FireAntsEvent.vi"("error in (no error)"=w444, "Ants in"=w443) -> ("error out"=w442:errorcluster)  [unwired: 2 in, 7 out]
                  n113 = call "Reset layer template selection.vi"("error in (no error)"=w442, "Data in"=w441) -> ("error out"=w440:errorcluster, "Data out"=w439:T2)  [unwired: 1 in, 7 out]
                  n114 = call "Escape.vi"("error in"=w440, "Data in"=w439) -> ("error out"=w437:errorcluster, "Data out"=w438:T2)  [unwired: 8 out]
                }
                frame "Delete" {
                  n115 = call "IsAntsRectValid.vi"("AntsRect"=w452) -> ("Valid?"=w459:bool, "Max. Rect size?"=w455:bool)  [unwired: 9 out]
                  n116 = case shown="True" w455 {
                    tunnel: w459 -> [_ _]
                    tunnel: w454 -> [w470 w474]
                    tunnel: [w469 w481] -> w457
                    tunnel: [w468 w482] -> w456
                    tunnel: w453 -> [w461 w472]
                    tunnel: w452 -> [_ w480]
                    frame False {
                      w467 = TRUE ("Delete Selected Area?")
                      n117 = call "PrepareTemporaryView.vi"("Delete Selected Area?"=w467, "error in (no error)"=w461, "Valid Selection?"=w467, "Data in"=w470) -> ("error out"=w464:errorcluster, "Highlighted?"=w465:bool, "All Layers out"=w466:refnum<class "Layer.lvclass">[], "Data out"=w462:T2, "#Active Layer"=w463:i32)  [unwired: 1 in, 2 out]
                      n118 = call "Selection_SetNewData.vi"("#Active Layer"=w463, "error in"=w464, "Highlighted?"=w465, "All Layers In"=w466, "Data in"=w462) -> ("error out"=w469:errorcluster, "Data out"=w468:T2)  [unwired: 1 in, 3 out]
                    }
                    frame True {
                      n119 = Unbundle By Name(w474) -> ("Class.Icon"=w479:refnum<class "Icon.lvclass">)
                      n120 = call-dynamic "GET_All User Layers.vi"("error in (no error)"=w472, "Icon.lvclass in"=w479) -> ("error out"=w478:errorcluster, "User Layer"=w475:refnum<class "Layer.lvclass">[])  [unwired: 7 in, 1 out]
                      n121 = Array Size(array=w475) -> (size(s)=w476:i32)
                      n122 = for {
                        N: w476 -> [_]
                        tunnel: [w483] -> w477 mode=indexing
                        i -> [w483]
                      }
                      n123 = call "Set active Layer programmatically.vi"("error in"=w478, "Active Layer []"=w477, "Data in"=w474) -> ("error out"=w471:errorcluster, "Data out"=w473:T2)  [unwired: 7 in]
                      n124 = call "DeleteLayer.vi"("error in"=w471, "AntsRect"=w480, "Data in"=w473) -> ("error out"=w481:errorcluster, "Data out"=w482:T2)  [unwired: 5 out]
                    }
                  }
                  n125 = call "Escape.vi"("error in"=w457, "Data in"=w456) -> ("error out"=w460:errorcluster, "Data out"=w458:T2)  [unwired: 8 out]
                }
              }
            }
          }
        }
        frame True {
          n126 = Unbundle By Name(w502) -> ("Support.AntsRect"=w484:T11, "Support.Action"=w489:T7, "Support.Mouse Down?"=w498:bool, "Support.Mouse inside icon?"=w499:bool, "Ref.Tools"=w504:refnum<vi>)
          n127 = Equal?(x=lveventtype."Key Repeat", y=w495) -> (x = y?=w493:bool)
          n128 = Equal?(x=lveventtype."Key Repeat?", y=w495) -> (x = y?=w494:bool)
          n129 = Or(x=w493, y=w494) -> (x .or. y?=w492:bool)
          n130 = case shown="\"Tool\"" w489 {
            tunnel: w504 -> [_ w576 w668]
            tunnel: w503 -> [w509 w575 w671]
            tunnel: w502 -> [w511 w574 w676]
            tunnel: [w508 w573 w675] -> w501
            tunnel: [w507 w572 w670] -> w500
            tunnel: w499 -> [_ w571 _]
            tunnel: w498 -> [_ w570 _]
            tunnel: w491 -> [_ w569 w673]
            tunnel: w490 -> [_ w568 w669]
            tunnel: w488 -> [w510 w566 w674]
            tunnel: [w506 w565 w672] -> w486
            tunnel: w485 -> [w505 w564 _]
            tunnel: w484 -> [_ w563 _]
            frame "Default", Default {
              n131 = case shown="\"X\", \"x\"" w510 {
                tunnel: w511 -> [w520 w547 w554 w561]
                tunnel: w509 -> [w519 w546 w556 w562]
                tunnel: [w517 w547 w548 w557] -> w508
                tunnel: [w514 w546 w555 w558] -> w507
                tunnel: [w518 _ w552 w559] -> w506
                tunnel: w505 -> [w512 _ _ _]
                frame "V", "v" {
                  # "Paste"
                  n132 = call "IE Read from Clipboard.vi"("error in"=w519, "Data in"=w520) -> ("error out"=w515:errorcluster, "Key Focus"=w518:bool, "Data out"=w516:T2, "Empty Clipboard string?"=w513:bool)  [unwired: 6 in]
                  n133 = case shown="True" w513 {
                    tunnel: [w523 w530] -> w517
                    tunnel: w516 -> [w522 w531]
                    tunnel: w515 -> [w521 w533]
                    tunnel: [w521 w527] -> w514
                    tunnel: w512 -> [_ w526]
                    frame False {
                      w525 = u32 111  # Invalid tool value
                      w524 = FALSE ("Support.CTRL Pressed")
                      n134 = Bundle By Name(cluster=w522, "Support.Shift pressed?"=w524, "Support.CTRL Pressed"=w524, "Support.Tool (old value)"=w525) -> (w523:T2)
                    }
                    frame True {
                      n135 = call "Empty Picture"() -> ("empty picture"=w534:picture)
                      n136 = call "Import_Clipboard.vi"("error in (no error)"=w533, "Picture in"=w534) -> ("error out"=w529:errorcluster, "Valid?"=w532:bool, "Picture"=w528:picture)  [unwired: 1 in, 6 out]
                      n137 = case shown="True" w532 {
                        tunnel: w531 -> [w536 w543]
                        tunnel: [w536 w539] -> w530
                        tunnel: w529 -> [w535 w544]
                        tunnel: w528 -> [_ w545]
                        tunnel: [w535 w538] -> w527
                        tunnel: w526 -> [_ w537]
                        frame False {
                        }
                        frame True {
                          n138 = call "Create new layer_LayerName_Picture.vi"("error in"=w544, "Layer name"=w537, "Picture"=w545, "Data in"=w543) -> ("error out"=w542:errorcluster, "Data out"=w541:T2)  [unwired: 6 in]
                          n139 = call "ViewLayer.vi"("Add to Undo?"=TRUE, "error in (no error)"=w542, "Data in"=w541) -> ("error out"=w538:errorcluster, "Data out"=w539:T2)  [unwired: 1 in, 6 out]
                        }
                      }
                    }
                  }
                }
                frame Default {
                }
                frame "C", "c" {
                  w551 = u32 111  # Invalid tool value
                  w550 = FALSE ("Support.CTRL Pressed")
                  n140 = call "IE Write to Clipboard.vi"("Is Cut?"=FALSE, "error in"=w556, "Data in"=w554) -> ("error out"=w555:errorcluster, "Key Focus"=w552:bool, "Data out"=w549:T2)  [unwired: 6 in]
                  n141 = Bundle By Name(cluster=w549, "Support.Shift pressed?"=w550, "Support.CTRL Pressed"=w550, "Support.Tool (old value)"=w551) -> (w548:T2)
                }
                frame "X", "x" {
                  n142 = call "IE Write to Clipboard.vi"("Is Cut?"=TRUE, "error in"=w562, "Data in"=w561) -> ("error out"=w558:errorcluster, "Key Focus"=w559:bool, "Data out"=w557:T2)  [unwired: 6 in]
                }
              }
            }
            frame "Tool" {
              n143 = Compound Arithmetic op=AND(invert w570, w571) -> (w567:bool)
              n144 = case shown="\"X\", \"x\"" w566 {
                tunnel: w576 -> [w589 _ _ _]
                tunnel: w575 -> [w588 w641 w659 w666]
                tunnel: w574 -> [w585 w645 w661 w667]
                tunnel: [w584 w643 w660 w662] -> w573
                tunnel: [w582 w644 w658 w664] -> w572
                tunnel: w567 -> [w581 _ _ _]
                tunnel: w569 -> [w580 _ _ _]
                tunnel: w568 -> [w579 _ _ _]
                tunnel: [_ w640 w656 w663] -> w565
                tunnel: w564 -> [_ w642 _ _]
                tunnel: w563 -> [w578 _ _ _]
                frame Default {
                  n145 = call "IsAntsRectValid.vi"("AntsRect"=w578) -> ("Valid?"=w577:bool)  [unwired: 10 out]
                  n146 = property class="RadioBtnsControl (strict)"(reference=w589, error in=w588) -> (reference out=w583:refnum<vi>, error out=w586:errorcluster, "Value"=w587:T12)
                  n147 = case shown="\"Select\"" w587 {
                    selector: w587 -> [w596 w615 _]
                    tunnel: w586 -> [w594 w618 w638]
                    tunnel: w585 -> [w598 w620 w639]
                    tunnel: [w597 w619 w637] -> w584
                    tunnel: w581 -> [w595 _ _]
                    tunnel: w583 -> [w593 w616 _]
                    tunnel: [w592 w617 w638] -> w582
                    tunnel: w580 -> [w591 w614 w636]
                    tunnel: w579 -> [w590 w613 w635]
                    tunnel: w577 -> [_ w621 _]
                    frame "Pencil", Default {
                      n148 = case shown="False" w595 {
                        tunnel: w598 -> [w603 w607]
                        tunnel: [w601 w612] -> w597
                        tunnel: w596 -> [_ w611]
                        tunnel: w594 -> [w602 w606]
                        tunnel: w593 -> [_ w610]
                        tunnel: [w602 w609] -> w592
                        tunnel: w591 -> [_ w605]
                        tunnel: w590 -> [_ w604]
                        frame False {
                          w600 = u32 111  # Invalid tool value
                          w599 = FALSE ("Support.CTRL Pressed")
                          n149 = Bundle By Name(cluster=w603, "Support.Shift pressed?"=w599, "Support.CTRL Pressed"=w599, "Support.Tool (old value)"=w600) -> (w601:T2)
                        }
                        frame True {
                          n150 = property class="RadioBtnsControl (strict)"(reference=w610, error in=w606, "Val(Sgnl)"=T12."Dropper" ("Value (Signaling)")) -> (error out=w609:errorcluster)  [unwired: 1 out]
                          n151 = Bundle By Name(cluster=w607, "Support.Tool (old value)"=w611, "Support.Shift pressed?"=w605, "Support.CTRL Pressed"=w604) -> (w612:T2)
                        }
                      }
                    }
                    frame "Select" {
                      n152 = case shown="True" w621 {
                        tunnel: w620 -> [w626 w634]
                        tunnel: [w625 w632] -> w619
                        tunnel: w618 -> [w629 w633]
                        tunnel: [w628 w633] -> w617
                        tunnel: w616 -> [w627 _]
                        tunnel: w615 -> [w624 _]
                        tunnel: w614 -> [w623 _]
                        tunnel: w613 -> [w622 _]
                        frame False {
                          n153 = Bundle By Name(cluster=w626, "Support.Tool (old value)"=w624, "Support.Shift pressed?"=w623, "Support.CTRL Pressed"=w622) -> (w625:T2)
                          n154 = property class="RadioBtnsControl (strict)"(reference=w627, error in=w629, "Val(Sgnl)"=T12."Dropper" ("Value (Signaling)")) -> (error out=w628:errorcluster)  [unwired: 1 out]
                        }
                        frame True {
                          w631 = u32 111  # Invalid tool value
                          n155 = Bundle By Name(cluster=w634, "Support.Tool (old value)"=w631) -> (w632:T2)
                        }
                      }
                    }
                    frame "Dropper" {
                      n156 = Bundle By Name(cluster=w639, "Support.Shift pressed?"=w636, "Support.CTRL Pressed"=w635) -> (w637:T2)
                    }
                  }
                }
                frame "V", "v" {
                  n157 = call "IE Read from Clipboard.vi"("error in"=w641, "Data in"=w645) -> ("error out"=w647:errorcluster, "Key Focus"=w640:bool, "Data out"=w648:T2, "Empty Clipboard string?"=w646:bool)  [unwired: 6 in]
                  n158 = case shown="False" w646 {
                    tunnel: [w651 w654] -> w643
                    tunnel: w648 -> [w650 w654]
                    tunnel: w647 -> [w649 w655]
                    tunnel: [w649 w655] -> w644
                    tunnel: w642 -> [_ _]
                    frame False {
                      w653 = u32 111  # Invalid tool value
                      w652 = FALSE ("Support.CTRL Pressed")
                      n159 = Bundle By Name(cluster=w650, "Support.Shift pressed?"=w652, "Support.CTRL Pressed"=w652, "Support.Tool (old value)"=w653) -> (w651:T2)
                    }
                    frame True {
                    }
                  }
                }
                frame "C", "c" {
                  n160 = call "IE Write to Clipboard.vi"("Is Cut?"=FALSE, "error in"=w659, "Data in"=w661) -> ("error out"=w658:errorcluster, "Key Focus"=w656:bool, "Data out"=w660:T2)  [unwired: 6 in]
                }
                frame "X", "x" {
                  n161 = call "IE Write to Clipboard.vi"("Is Cut?"=TRUE, "error in"=w666, "Data in"=w667) -> ("error out"=w664:errorcluster, "Key Focus"=w663:bool, "Data out"=w662:T2)  [unwired: 6 in]
                }
              }
            }
            frame "Move Selection" {
              n162 = case shown="\"Z\", \"z\"" w674 {
                tunnel: w671 -> [w677 w684 w696]
                tunnel: w676 -> [w678 w683 w697]
                tunnel: [w678 w682 w694] -> w675
                tunnel: w673 -> [_ w681 _]
                tunnel: [_ w680 _] -> w672
                tunnel: [w677 w679 w695] -> w670
                tunnel: w669 -> [_ _ _]
                tunnel: w668 -> [_ _ _]
                frame Default {
                }
                frame "Z", "z" {
                  n163 = case shown="False" w681 {
                    tunnel: w684 -> [w688 w691]
                    tunnel: w683 -> [w690 w693]
                    tunnel: [w689 w693] -> w682
                    tunnel: [TRUE TRUE] -> w680
                    tunnel: [w687 w691] -> w679
                    frame False {
                      n164 = call "Escape.vi"("Reset cursor (T)"=FALSE, "error in"=w688, "Data in"=w690) -> ("error out"=w687:errorcluster, "Data out"=w689:T2)  [unwired: 7 out]
                    }
                    frame True {
                    }
                  }
                }
                frame "V", "v" {
                  n165 = call "Finalize Movement.vi"("error in (no error)"=w696, "Data in"=w697) -> ("error out"=w695:errorcluster, "Data out"=w694:T2)  [unwired: 2 in, 6 out]
                }
              }
            }
          }
          n166 = Or(x=w486, y=w492) -> (x .or. y?=w487:bool)
        }
      }
    }
    frame Error {
    }
  }
  "error out" <- w9
  "Discard?" <- w5
  "Data out" <- w3
